vi "Configure Median Filter.vi"(7 "Median Rank (1 Rank1)":i32(ring)=1 items=["Rank1"=1, "Rank2"=2, "Rank3"=3, "Rank4"=4, "Rank5"=5], 8 "error in (no error)":errorcluster, 9 "Enable Median Filter (T: Enable)":bool=TRUE, 10 "Measurement Function (0: Voltage)":i32(ring) items=["Voltage", "Current", "Resistance", "Charge"], 11 "VISA resource name":refnum<visa-resource-name>) -> (0 "error out":errorcluster, 3 "VISA resource name out":refnum<visa-resource-name>)   [LabVIEW 2019, in "Keithley 6517.lvlib"]
doc: "Enables or disables the median filter, and configures the median rank for the measurement functions (Voltage, Current, Resistance and Charge).\n\nNote:\n(1) The specified measurement should be enabled from <b>Configure Measurement Function.vi</b>.\n(2) <B>Measurement Function</B> control is NOT compatible with <B>modoel 6514</B> (changing this setting will not affect the instrument)."
uses:
  Keithley 6517.lvlib
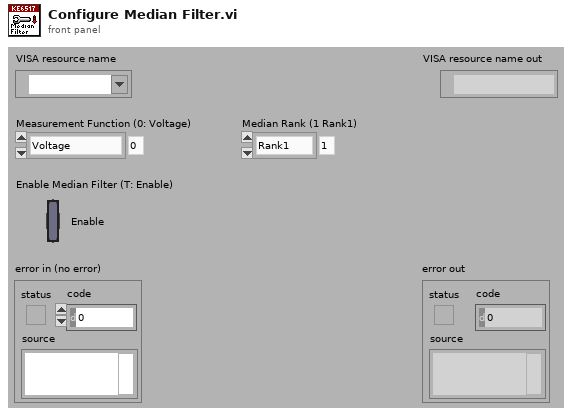
[diagram p1: front panel]
types:
  T1 = typedef "Keithley 6517.lvlib/Extended User Data.ctl" = cluster{"Instrument Model":i32}
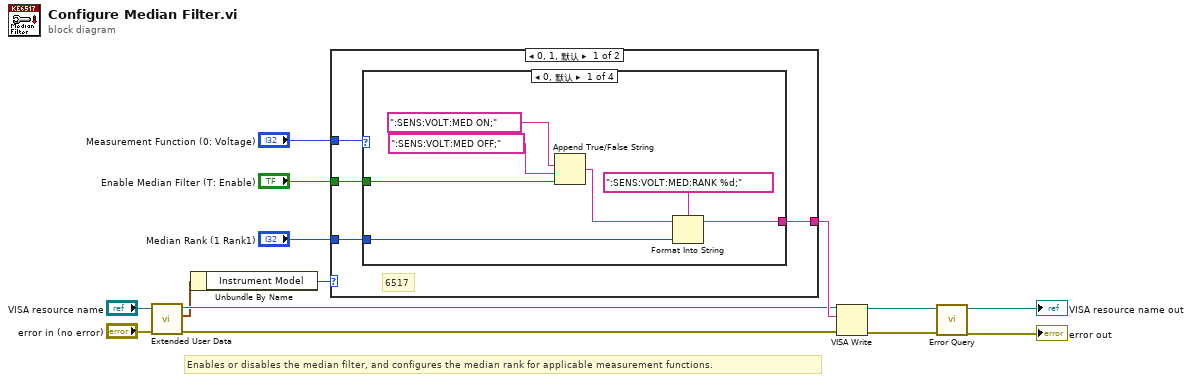
[diagram p0: block diagram]
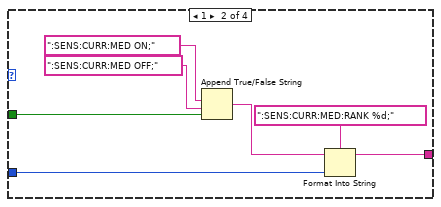
[diagram p2: hidden frame]
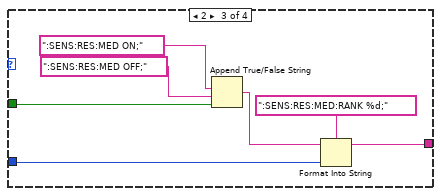
[diagram p3: hidden frame]
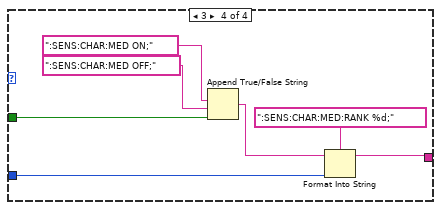
[diagram p4: hidden frame]
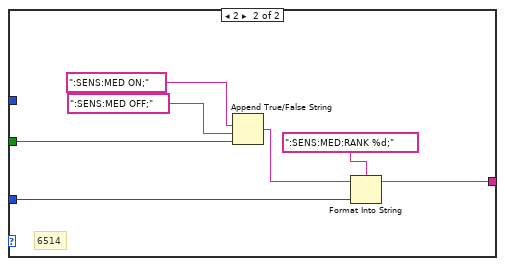
[diagram p5: hidden frame]
diagram:
  # "Enables or disables the median filter, and configures the median rank for applicable measurement functions."
  n1 = call "Extended User Data.vi"("error in (no error)"="error in (no error)", "VISA resource name"="VISA resource name") -> ("error out"=w3:errorcluster, "User Data Out"=w2:T1, "VISA resource name out"=w4:refnum<visa-resource-name>)  [unwired: 7 in]
  n2 = Unbundle By Name(w2) -> ("Instrument Model"=w1:i32)
  n3 = case shown="0, 1, 默认" w1 {
    tunnel: "Enable Median Filter (T: Enable)" -> [w18 w53]
    tunnel: "Median Rank (1 Rank1)" -> [w17 w52]
    tunnel: [w16 w51] -> w8
    tunnel: "Measurement Function (0: Voltage)" -> [w15 _]
    frame 0, 1, Default {
      # "6517"
      n4 = case shown="0, 默认" w15 {
        tunnel: w18 -> [w22 w28 w35 w42]
        tunnel: w17 -> [w21 w27 w34 w41]
        tunnel: [w19 w26 w33 w40] -> w16
        frame 0, Default {
          n5 = Append True/False String(1:w22, 2:":SENS:VOLT:MED OFF;", 3:":SENS:VOLT:MED ON;") -> (0:w24:string)  [unwired: 1 in]
          n6 = Format Into String(format string=":SENS:VOLT:MED:RANK %d;", initial string=w24, w21) -> (resulting string=w19:string)  [unwired: 1 in, 1 out]
        }
        frame 1 {
          n7 = Append True/False String(1:w28, 2:":SENS:CURR:MED OFF;", 3:":SENS:CURR:MED ON;") -> (0:w32:string)  [unwired: 1 in]
          n8 = Format Into String(format string=":SENS:CURR:MED:RANK %d;", initial string=w32, w27) -> (resulting string=w26:string)  [unwired: 1 in, 1 out]
        }
        frame 2 {
          n9 = Append True/False String(1:w35, 2:":SENS:RES:MED OFF;", 3:":SENS:RES:MED ON;") -> (0:w39:string)  [unwired: 1 in]
          n10 = Format Into String(format string=":SENS:RES:MED:RANK %d;", initial string=w39, w34) -> (resulting string=w33:string)  [unwired: 1 in, 1 out]
        }
        frame 3 {
          n11 = Append True/False String(1:w42, 2:":SENS:CHAR:MED OFF;", 3:":SENS:CHAR:MED ON;") -> (0:w45:string)  [unwired: 1 in]
          n12 = Format Into String(format string=":SENS:CHAR:MED:RANK %d;", initial string=w45, w41) -> (resulting string=w40:string)  [unwired: 1 in, 1 out]
        }
      }
    }
    frame 2 {
      # "6514"
      n13 = Append True/False String(1:w53, 2:":SENS:MED OFF;", 3:":SENS:MED ON;") -> (0:w49:string)  [unwired: 1 in]
      n14 = Format Into String(format string=":SENS:MED:RANK %d;", initial string=w49, w52) -> (resulting string=w51:string)  [unwired: 1 in, 1 out]
    }
  }
  n15 = VISA Write(VISA resource name=w4, write buffer=w8, error in (no error)=w3) -> (VISA resource name out=w14:refnum<visa-resource-name>, error out=w13:errorcluster)  [unwired: 1 out]
  n16 = call "Error Query.vi"("error in (no error)"=w13, "VISA resource name"=w14) -> ("error out"=→"error out":errorcluster, "VISA resource name out"=→"VISA resource name out":refnum<visa-resource-name>)  [unwired: 6 in, 2 out]
